vi "Cond Timed Wait (absolute timespec).vi"(8 "error in (no error)":errorcluster, 9 "absolute timeout (timespec)":T1, 10 "Mutex in":T2, 11 "Cond in":T3) -> (0 "error out":errorcluster, 1 "timed out?":bool, 2 "Mutex out":T2, 3 "Cond out":T3)   [LabVIEW 2013, in "POSIX Threads.lvlib" / "Cond.lvclass"]
doc: "Calls pthread_cond_timedwait() on the pthread cond object encapsulated by Cond.\n\nTo provide a valid absolute timeout, query the appropriate clock for the current time and offset the time by the desired timeout duration. By default, conditional variables use the Realtime clock when evaluating the absolute timeout, but this clock can be changed using the Cond attribute, Set Clock.\n\nRefer to online POSIX documentation for more information."
uses:
  Cond.lvclass
  Controls/reference.ctl
  Mutex/Controls/reference.ctl
  Mutex/Mutex.lvclass
  <vilib>/NI/NI Linux RT Utilities/Controls/Public/C Structs/timespec_64.ctl
  POSIX Thread Object/POSIX Thread Object.lvclass/POSIX Thread Object.ctl
  POSIX Thread Object/Private VIs/libpthread path.vi
  <vilib>/NI/NI Linux RT Utilities/VIs/Public/Convert Types/convert timespec 64 to timespec 32.vi
  POSIX Thread Object/Private VIs/get pthread error.vi
  POSIX Thread Object/POSIX Thread Object.lvclass
  <vilib>/NI/NI Linux RT Utilities/Linux RT Utilities.lvlib
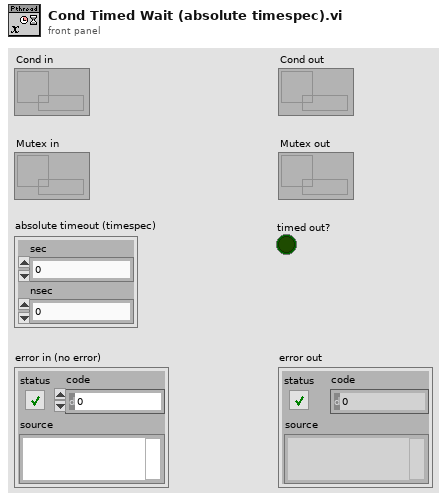
[diagram p1: front panel]
types:
  T1 = typedef "Linux RT Utilities.lvlib/timespec_64.ctl" = cluster{"sec":u64, "nsec":u64}
  T2 = typedef "POSIX Threads.lvlib/Mutex.lvclass/reference.ctl" = refnum<data-value>
  T3 = typedef "POSIX Threads.lvlib/Cond.lvclass/reference.ctl" = refnum<data-value>
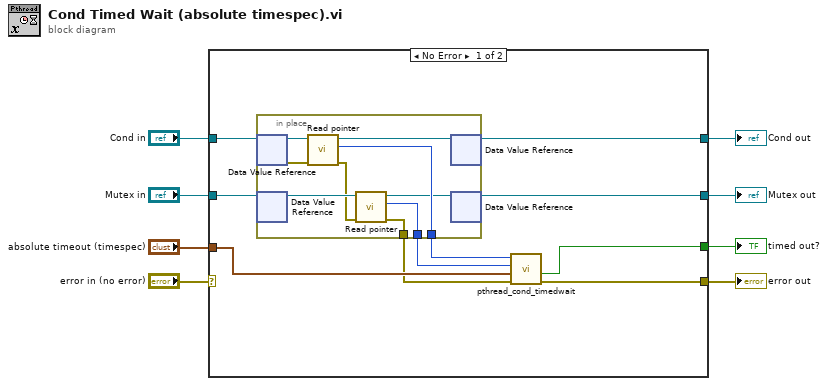
[diagram p0: block diagram]
diagram:
  n1 = case shown="No Error" "error in (no error)" {
    selector: "error in (no error)" -> [_ w30]
    tunnel: [w18 w30] -> w7
    tunnel: "Cond in" -> [w15 w29]
    tunnel: [w14 w29] -> w5
    tunnel: "Mutex in" -> [w13 w28]
    tunnel: [w9 w28] -> w3
    tunnel: "absolute timeout (timespec)" -> [w16 _]
    tunnel: [w17 _] -> w1
    frame No Error {
      n2 = in-place {
        in-place-border: [w24] -> w10
        in-place-border: [w20] -> w12
        in-place-border: [w19] -> w11
        n3 = in-place-dvr #1(w15) -> (w27:refnum<class "Cond.lvclass">, w25:errorcluster)
        n4 = in-place-dvr #2(w13) -> (w23:refnum<class "Mutex.lvclass">)  [unwired: 1 out]
        n5 = call "Read pointer.vi"("error in (no error)"=w25, "POSIX Thread Object in"=w27) -> ("error out"=w21:errorcluster, "pointer"=w24:u64, "POSIX Thread Object out"=w26:refnum<class "Cond.lvclass">)  [unwired: 7 in]
        n6 = call "Read pointer.vi"("error in (no error)"=w21, "POSIX Thread Object in"=w23) -> ("error out"=w20:errorcluster, "pointer"=w19:u64, "POSIX Thread Object out"=w22:refnum<class "Mutex.lvclass">)  [unwired: 7 in]
        n7 = in-place-dvr #1(w26) -> (w14:T3)  [unwired: 1 out]
        n8 = in-place-dvr #2(w22) -> (w9:T2)  [unwired: 1 out]
      }
      n9 = call "pthread_cond_timedwait.vi"("error in (no error)"=w12, "absolute time"=w16, "mutex ptr in"=w11, "cond ptr in"=w10) -> ("error out"=w18:errorcluster, "timed out?"=w17:bool)  [unwired: 4 in, 2 out]
    }
    frame Error {
    }
  }
  "Cond out" <- w5
  "error out" <- w7
  "Mutex out" <- w3
  "timed out?" <- w1
